vi "CL_Evaluate Analog PID.vi"(8 "error in":errorcluster, 11 "PID Tag Sets":T2[](array[typedef])) -> (0 "error out":errorcluster, 1 "PID Loop Errors":dbl[](array[numeric]), 3 "PID Control Outputs":dbl[](array[numeric]), 5 "PID_Parameters":T1[](array[typedef])=[{"Set Point (%)"=0.0, "PID_Gains"={"proportional gain (Kc)"=1.0, "integral time (Ti, min)"=0.01, "derivative time (Td, min)"=0.0}, "PID_Output_Range"={"OUTHI"=100.0, "OUTLO"=0.0}, "Mode"=FALSE, "Manual Value"=1.0, "PID_OK?"=FALSE, "Setpoint_Range"={"setpoint low"=0.0, "setpoint hi"=100.0}}] {"Setpoint_Range"."setpoint low" format="%.2f"; "Setpoint_Range"."setpoint hi" format="%.2f"; "Manual Value" format="%.3f"; "Set Point (%)" scale=0.0..100.0; "PID_Output_Range"."OUTLO" format="%.2f"; "PID_Output_Range"."OUTHI" format="%.2f"; "PID_Gains"."derivative time (Td, min)" format="%.3f"; "PID_Gains"."integral time (Ti, min)" format="%.3f"; "PID_Gains"."proportional gain (Kc)" format="%.3f"})   [LabVIEW 2010]
doc: "NGTS array based PID evaluation. PID Tag values are formated into arrays of parameters for NI PID VIs. Outputs.\n\n2007 Mike Ashe\nmichael.ashe@imaginatics.net\nCell: 860-961-0876"
uses:
  <vilib>/addons/control/pid/NI_PID_pid.lvlib
  SmartBuffer_DBL/Public TypeDefs/SB_Operation Method.ctl
  Controls/NGTS_PID Loop Tag and Gain Set.ctl
  PID_Parameters_TT.ctl
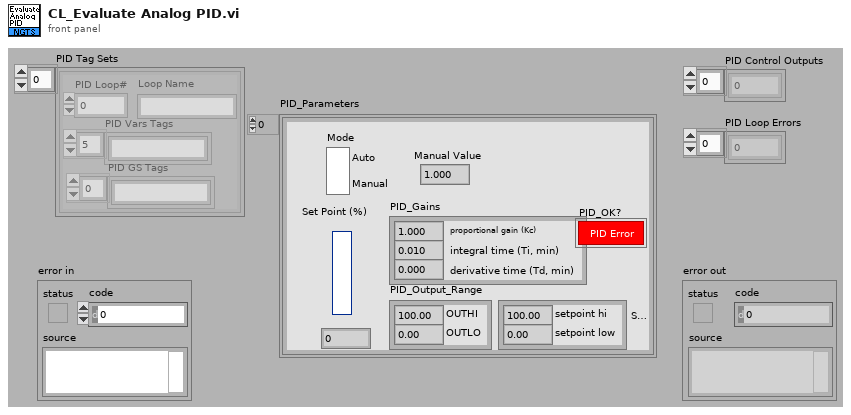
[diagram p1: front panel]
types:
  T1 = typedef "PID_Parameters_TT.ctl" = cluster{"Set Point (%)":dbl, "PID_Gains":cluster{"proportional gain (Kc)":dbl, "integral time (Ti, min)":dbl, "derivative time (Td, min)":dbl}, "PID_Output_Range":cluster{"OUTHI":dbl, "OUTLO":dbl}, "Mode":bool, "Manual Value":dbl, "PID_OK?":bool, "Setpoint_Range":cluster{"setpoint low":dbl, "setpoint hi":dbl}}
  T2 = typedef "NGTS_PID Loop Tag and Gain Set.ctl" = cluster{"PID Loop#":i32, "PID Vars Tags":string[], "PID GS Tags":string[], "Loop Name":string}
  T3 = typedef "SmartBuffer_DBL.lvlib/SB_Operation Method.ctl" = enum16{"initialize", "register read op", "read data", "read data by tags", "register write op", "write data", "write data by tags", "import buffer image", "export buffer image", "register/replace read op", "register/replace write op"}
  T4 = typedef "SmartBuffer_DBL.lvlib/SB_Control_TypeDef.ctl" = dbl
  T5 = cluster{"PID gains":cluster{"proportional gain (Kc)":dbl, "integral time (Ti, min)":dbl, "derivative time (Td, min)":dbl}, "max value":dbl}[]
  T6 = cluster{"proportional gain (Kc)":dbl, "integral time (Ti, min)":dbl, "derivative time (Td, min)":dbl}
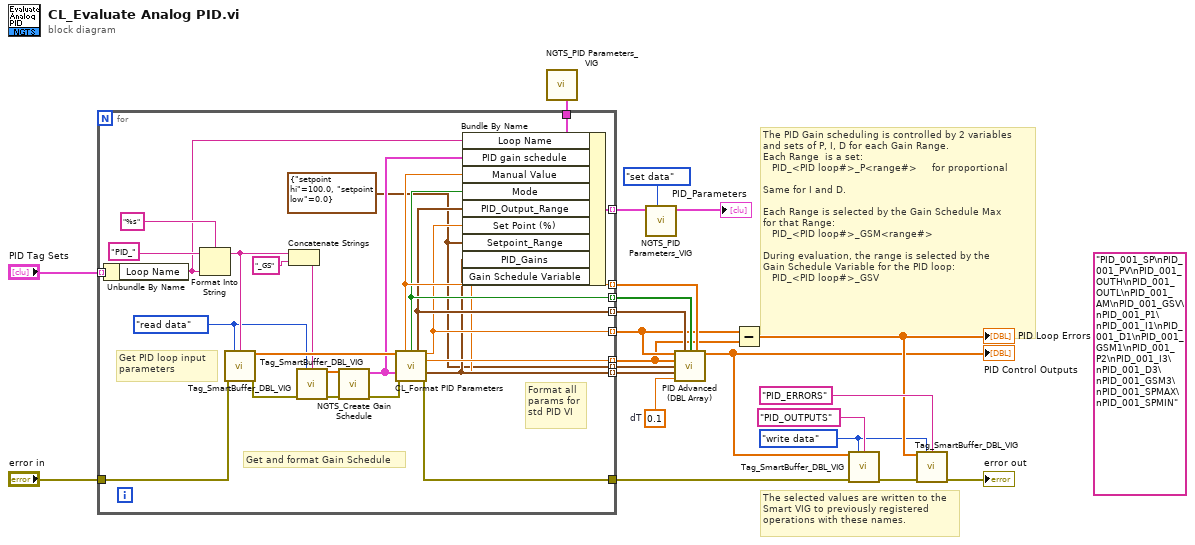
[diagram p0: block diagram]
diagram:
  w1 = SB_Operation_Method."write data" ("SmartBuffer_Method")
  w19 = 0.1  # dT
  (unwired) "PID_001_SP\nPID_001_PV\nPID_001_OUTH\nPID_001_OUTL\nPID_001_AM\nPID_001_GSV\nPID_001_P1\nPID_001_I1\nPID_001_D1\nPID_001_GSM1\nPID_001_P2\nPID_001_I3\nPID_001_D3\nPID_001_GSM3\nPID_001_SPMAX\nPID_001_SPMIN"
  # "The PID Gain scheduling is controlled by 2 variables\nand sets of P, I, D for each Gain Range.\nEach Range  is a set:\n   PID_<PID loop#>_P<range#>     for proportional\n\nSame for I and D.\n\nEach Range is selected by the Gain Schedule Max\nfor that Range:\n   PID_<PID loop#>_GSM<range#>\n\nDuring evaluation, the range is selected by the\nGain Schedule Variable for the PID loop:\n   PID_<PID loop#>_GSV"
  # "The selected values are written to the\nSmart VIG to previously registered\noperations with these names."
  n1 = call "NGTS_PID Parameters_VIG.vi"() -> ("PID Param (Blank)"=w5:T1)  [unwired: 9 in, 2 out]
  n2 = for {
    tunnel: "error in" -> [w47]
    tunnel: [w43] -> w10
    tunnel: [w28] -> w15 mode=indexing
    tunnel: [w44] -> w7 mode=indexing
    tunnel: [w24] -> w21 mode=indexing
    tunnel: [w26] -> w20 mode=indexing
    tunnel: [w29] -> w18 mode=indexing
    tunnel: [w30] -> w17 mode=indexing
    tunnel: [w32] -> w16 mode=indexing
    tunnel: "PID Tag Sets" -> [w42] mode=indexing
    tunnel: w5 -> [w33]
    tunnel: [w27] -> w4 mode=indexing
    w24 = cluster{"setpoint hi":dbl, "setpoint low":dbl} {"setpoint hi"=100.0, "setpoint low"=0.0} ("Setpoint_Range")
    w37 = SB_Operation_Method."read data" ("SmartBuffer_Method")
    # "Get and format Gain Schedule"
    # "Format all\nparams for\nstd PID VI"
    # "Get PID loop input\nparameters"
    n3 = Unbundle By Name(w42) -> ("Loop Name"=w23:string)
    n4 = Format Into String(format string="%s", initial string="PID_" ("TagOp_Name"), w23) -> (resulting string=w41:string)  [unwired: 1 in, 1 out]
    n5 = call "Tag_SmartBuffer_DBL_VIG.vi"("SmartBuffer_Method"=w37, "TagOp_Name"=w41, "error in"=w47) -> ("tag_data_out"=w45:T4[], "error out"=w38:errorcluster)  [unwired: 6 in, 5 out]
    n6 = Concatenate Strings(w41, "_GS" ("string")) -> (w39:string)
    n7 = call "Tag_SmartBuffer_DBL_VIG.vi"("SmartBuffer_Method"=w37, "TagOp_Name"=w39, "error in"=w38) -> ("tag_data_out"=w34:T4[], "error out"=w36:errorcluster)  [unwired: 6 in, 5 out]
    n8 = call "NGTS_Create Gain Schedule.vi"("error in"=w36, "tag_data_in"=w34) -> ("error out"=w35:errorcluster, "PID gain schedule"=w31:T5)  [unwired: 8 in]
    n9 = call "CL_Format PID Parameters.vi"("PID Cfg"=w45, "PID gain schedule"=w31, "error in"=w35) -> ("Manual"=w32:dbl, "Mode"=w30:bool, "output range"=w29:cluster{"output high":dbl, "output low":dbl}, "Setpoint"=w28:dbl, "Process Variable"=w44:dbl, "PID gains out"=w26:T6, "Gain Schedule Variable"=w25:dbl, "error out"=w43:errorcluster)  [unwired: 5 in]
    n10 = Bundle By Name(cluster=w33, "Loop Name"=w23, "PID gain schedule"=w31, "Manual Value"=w32, "Mode"=w30, "PID_Output_Range"=w29, "Set Point (%)"=w28, "Setpoint_Range"=w24, "PID_Gains"=w26, "Gain Schedule Variable"=w25) -> (w27:T1)
  }
  n11 = call "NGTS_PID Parameters_VIG.vi"("Operation"=enum16{"get data", "set data", "initialize"}."set data", "PID_Parameters In"=w4) -> ("PID_Parameters Out"=→"PID_Parameters":T1[])  [unwired: 7 in, 2 out]
  n12 = call <vilib>:"PID Advanced (DBL Array).vi"("setpoint"=w15, "output range"=w18, "auto? (T)"=w17, "manual control"=w16, "process variable"=w7, "setpoint range"=w21, "PID gains"=w20, "dt (s)"=w19) -> ("output"=w11:dbl[])  [unwired: 6 in, 1 out]
  "PID Control Outputs" <- w11
  n13 = Subtract(x=w15, y=w7) -> (x-y=w12:dbl[])
  "PID Loop Errors" <- w12
  n14 = call "Tag_SmartBuffer_DBL_VIG.vi"("tag_data_in"=w11, "SmartBuffer_Method"=w1, "TagOp_Name"="PID_OUTPUTS", "error in"=w10) -> ("error out"=w9:errorcluster)  [unwired: 5 in, 6 out]
  n15 = call "Tag_SmartBuffer_DBL_VIG.vi"("tag_data_in"=w12, "SmartBuffer_Method"=w1, "TagOp_Name"="PID_ERRORS", "error in"=w9) -> ("error out"=→"error out":errorcluster)  [unwired: 5 in, 6 out]
